vi "TEST Object Manual Bounds (Viewport).vi"() -> ()   [LabVIEW 2021, in "IObject.lvclass"]
uses:
  IObject.lvclass
  <vilib>/Utility/miscctls.llb/LVRectTypeDef.ctl
  Object/Object.lvclass
  C:/Projects/Dynamic-Scaling/Dynamic Scaling/IObject.lvclass
  IContainer/Viewport/Viewport.lvclass
panel:
  in  "OK Button 2":dbl(graph)
  in  "Bounds":T1={"Left"=100, "Top"=50, "Right"=400, "Bottom"=250}
  in  "OK Button 1":bool
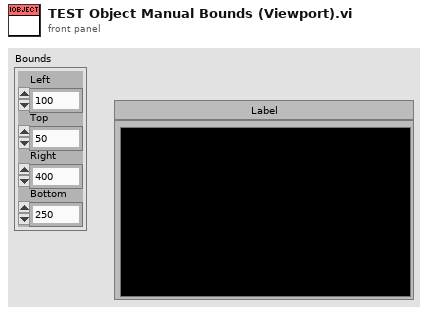
[diagram p1: front panel]
types:
  T1 = typedef "LVRectTypeDef.ctl" = cluster{"Left":i16, "Top":i16, "Right":i16, "Bottom":i16}
  T2 = cluster{"Left":dbl, "Top":dbl, "Right":dbl, "Bottom":dbl}[]
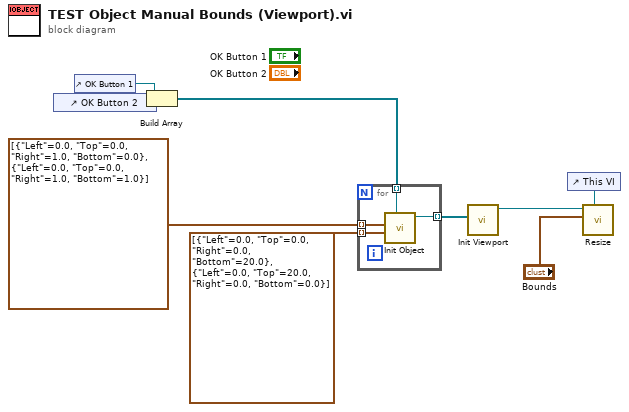
[diagram p0: block diagram]
diagram:
  n1 = control-ref of="OK Button 2"() -> (w8:refnum<vi>)
  n2 = control-ref of="OK Button 1"() -> (w9:refnum<vi>)
  n3 = Build Array(w9, w8) -> (w7:refnum<vi>[])
  n4 = for {
    tunnel: T2 [{"Left"=0.0, "Top"=0.0, "Right"=1.0, "Bottom"=0.0}, {"Left"=0.0, "Top"=0.0, "Right"=1.0, "Bottom"=1.0}] -> [w13] mode=indexing
    tunnel: w7 -> [w12] mode=indexing
    tunnel: T2 [{"Left"=0.0, "Top"=0.0, "Right"=0.0, "Bottom"=20.0}, {"Left"=0.0, "Top"=20.0, "Right"=0.0, "Bottom"=0.0}] -> [w11] mode=indexing
    tunnel: [w10] -> w3 mode=indexing
    n5 = call "Init Object.vi"("GObj Refnum"=w12, "B [0, 0, 0, 0]"=w11, "A [0, 0, 1, 1]"=w13) -> ("MMI Scaling out"=w10:refnum<class "Object.lvclass">)  [unwired: 7 in, 1 out]
  }
  n6 = call "Init Viewport.vi"("Items"=w3) -> ("Viewport out"=w2:refnum<class "Viewport.lvclass">)  [unwired: 9 in, 1 out]
  n7 = control-ref of="This VI"() -> (w4:refnum<vi>)
  n8 = call-dynamic "Resize.vi"("VI Refnum"=w4, "Bounds"="Bounds", "MMI Scaling in"=w2) -> ()  [unwired: 6 in, 3 out]
